vi "Flush Inbox.vi"(8 "error in":errorcluster, 11 "Messaging Manager Actor in":refnum<class "Messaging Manager Actor.lvclass">) -> (0 "error out":errorcluster, 3 "Messaging Manager Actor out":refnum<class "Messaging Manager Actor.lvclass">)   [LabVIEW 2024, in "PCAN.lvlib" / "Messaging Manager Actor.lvlib" / "Messaging Manager Actor.lvclass"]
uses:
  Messaging Manager Actor.lvclass
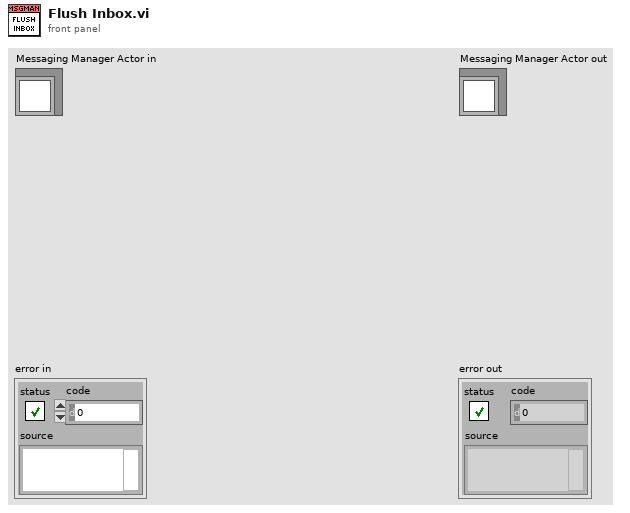
[diagram p1: front panel]
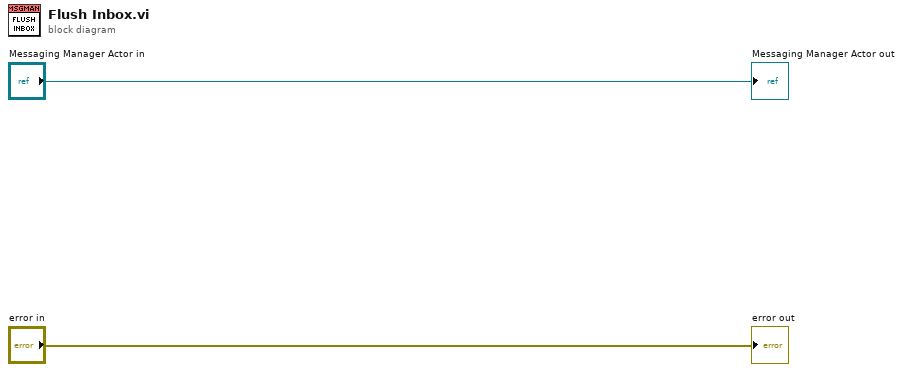
[diagram p0: block diagram]
diagram:
  "error out" <- "error in"
  "Messaging Manager Actor out" <- "Messaging Manager Actor in"
